vi "ev b index.vi"(8 "error in (no error)":errorcluster, 11 "IDE simple in":refnum<class "Main Panel.lvclass">) -> (0 "error out":errorcluster, 3 "IDE simple out":refnum<class "Main Panel.lvclass">)   [LabVIEW 2018, in "Main Panel.lvlib" / "Main Panel.lvclass"]
uses:
  Main Panel.lvclass
  Main Panel.lvclass/Main Panel.ctl
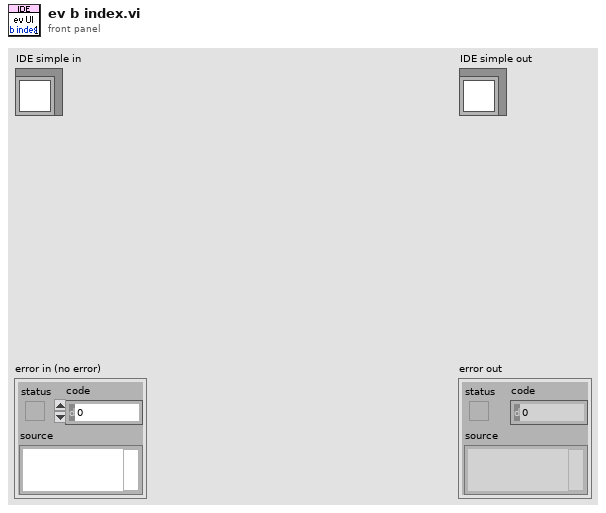
[diagram p1: front panel]
types:
  T1 = typedef "Data Parser.lvclass/frame b data.ctl" = cluster{"kind":string, "x":string, "y":string, "w":string, "h":string}
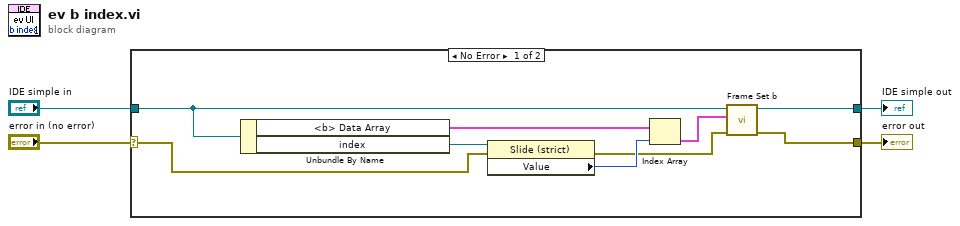
[diagram p0: block diagram]
diagram:
  n1 = case shown="No Error" "error in (no error)" {
    selector: "error in (no error)" -> [w5 w15]
    tunnel: [w7 w15] -> w3
    tunnel: [w6 w14] -> w1
    tunnel: "IDE simple in" -> [w12 w14]
    frame No Error {
      n2 = Unbundle By Name(w12) -> ("<b> Data Array"=w11:T1[], "index"=w13:refnum<vi>)
      n3 = property class="Slide (strict)"(reference=w13, error in=w5) -> (error out=w8:errorcluster, "Value"=w10:u32)  [unwired: 1 out]
      n4 = Index Array(array=w11, index=w10) -> (element=w9:T1)
      n5 = call "Frame Set b.vi"("error in (no error)"=w8, "<b> Data"=w9, "IDE simple in"=w12) -> ("error out"=w7:errorcluster, "IDE simple out"=w6:refnum<class "Main Panel.lvclass">)  [unwired: 7 in]
    }
    frame Error {
    }
  }
  "error out" <- w3
  "IDE simple out" <- w1
